vi "Init_Channels.vi"(8 "Error in":errorcluster, 11 "Channel_Information":T1 {"Input Terminal Configuration" items=["default"=-1, "RSE"=10083, "NRSE"=10078, "Differential"=10106, "Pseudodifferential"=12529]}) -> (0 "Error Out":errorcluster, 3 "Task out":refnum<k21>)   [LabVIEW 2017]
doc: "Initiliaze Channels based on the specified Channel Type in the Channel Information Control"
uses:
  <vilib>/DAQmx/create/channels.llb/DAQmx Create Channel (AI-Current-Basic).vi
  <vilib>/DAQmx/create/channels.llb/DAQmx Create Channel (AI-Voltage-Basic).vi
  typedef/Channel_Information_Control_array.ctl
  typedef/Channel_Information_Control_single.ctl
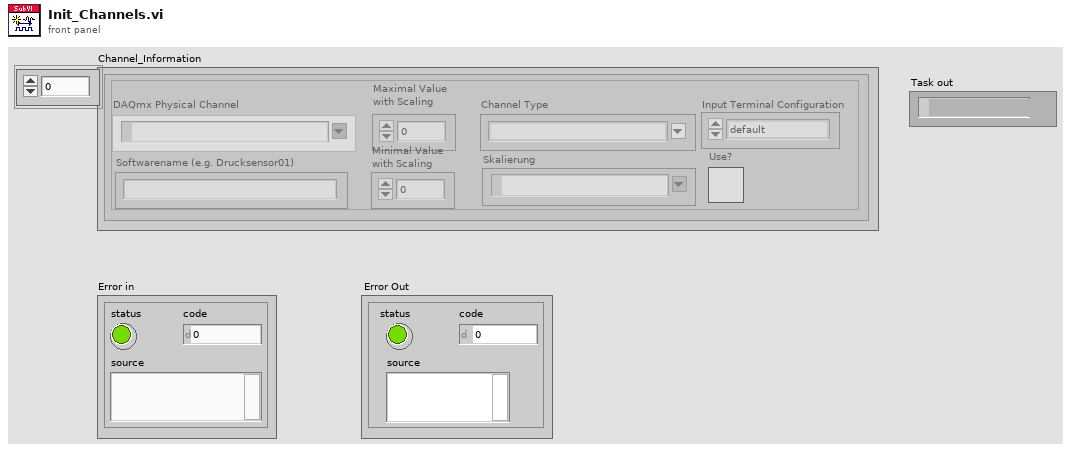
[diagram p1: front panel]
types:
  T1 = typedef "Channel_Information_Control_array.ctl" = T2[]
  T2 = typedef "Channel_Information_Control_single.ctl" = cluster{"DAQmx Physical Channel":tag, "Softwarename (e.g. Drucksensor01)":string, "Maximal Value \nwith Scaling":dbl, "Minimal Value\nwith Scaling":dbl, "Channel Type":string, "Input Terminal Configuration":i32, "Skalierung":tag, "Use?":bool}
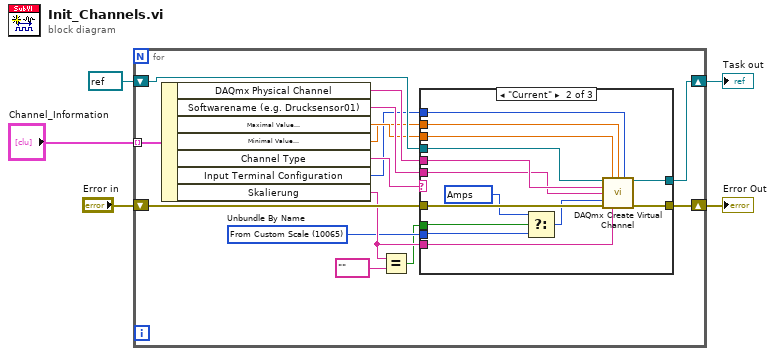
[diagram p0: block diagram]
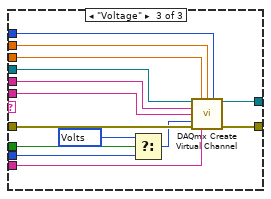
[diagram p3: hidden frame]
diagram:
  n1 = for {
    tunnel: "Channel_Information" -> [w20] mode=indexing
    shift-right: [w17] -> w3
    shift-left: refnum<k21> refnum ("task in") -> [w18]
    shift-right: [w11] -> w2
    shift-left: "Error in" -> [w10]
    w7 = 10065 items=["Volts"=10348, "From Custom Scale"=10065] ("units")
    n2 = Unbundle By Name(w20) -> ("DAQmx Physical Channel"=w16:tag, "Softwarename (e.g. Drucksensor01)"=w15:string, "Maximal Value \nwith Scaling"=w14:dbl, "Minimal Value\nwith Scaling"=w13:dbl, "Channel Type"=w19:string, "Input Terminal Configuration"=w12:i32, "Skalierung"=w9:tag)
    n3 = Equal?(x=w9, y=tag "") -> (x = y?=w6:bool)
    n4 = case shown="\"Current\"" w19 {
      tunnel: w18 -> [w22 w36 w50]
      tunnel: [w22 w29 w49] -> w17
      tunnel: w16 -> [_ w35 w48]
      tunnel: w15 -> [_ w34 w47]
      tunnel: w14 -> [_ w33 w46]
      tunnel: w13 -> [_ w32 w45]
      tunnel: w12 -> [_ w31 w44]
      tunnel: w9 -> [_ w30 w43]
      tunnel: [w21 w28 w42] -> w11
      tunnel: w10 -> [w21 w27 w41]
      tunnel: w7 -> [_ w25 w40]
      tunnel: w6 -> [_ w26 w39]
      frame Default {
      }
      frame "Current" {
        w24 = 10342 items=["Amps"=10342, "From Custom Scale"=10065] ("units")
        n5 = Select(t=w24, s=w26, f=w25) -> (s? t:f=w23:i32)
        n6 = call-poly <vilib>:"DAQmx Create Virtual Channel.vi"("task in"=w36, "maximum value"=w33, "minimum value"=w32, "input terminal configuration"=w31, "physical channels"=w35, "name to assign"=w34, "units"=w23, "error in"=w27, "custom scale name"=w30) -> ("task out"=w29:refnum<k21>, "error out"=w28:errorcluster)  [unwired: 5 in]
      }
      frame "Voltage" {
        w38 = 10348 items=["Volts"=10348, "From Custom Scale"=10065] ("units")
        n7 = Select(t=w38, s=w39, f=w40) -> (s? t:f=w37:i32)
        n8 = call-poly <vilib>:"DAQmx Create Virtual Channel.vi"("task in"=w50, "maximum value"=w46, "minimum value"=w45, "input terminal configuration"=w44, "physical channels"=w48, "name to assign"=w47, "units"=w37, "error in"=w41, "custom scale name"=w43) -> ("task out"=w49:refnum<k21>, "error out"=w42:errorcluster)  [unwired: 5 in]
      }
    }
  }
  "Task out" <- w3
  "Error Out" <- w2
